vi "Do.vi"(8 "error in (no error)":errorcluster, 10 "Actor in":refnum<class "Actor.lvclass">, 11 "Trace Query Options Msg":refnum<class "Trace Query Options Msg.lvclass">) -> (0 "error out":errorcluster, 2 "Actor out":refnum<class "Actor.lvclass">)   [LabVIEW 2017, in "BNT_DSCXtGraph.lvlib" / "Trace Query Options Msg.lvclass"]
doc: "This VI delivers the message to the actor by calling the appropriate method(s) on the actor."
uses:
  Trace Query Options Msg.lvclass
  <vilib>/ActorFramework/Actor/Actor.lvclass
  BNT_DSCXtGraph/BNT_DSCXtGraph.lvclass
  C:/Program Files (x86)/National Instruments/LabVIEW 2017/vi.lib/ActorFramework/Actor/Actor.lvclass
  Trace Query Options Msg.lvclass/Trace Query Options Msg.ctl
  CSPP_Core/Messages/CSPP_AsyncCallbackMsg/CSPP_AsyncCallback Msg.lvclass
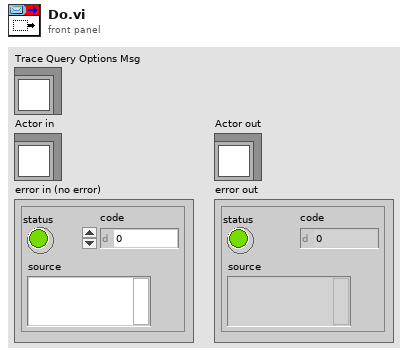
[diagram p1: front panel]
types:
  T1 = cluster{"Start Time":timestamp, "Stop Time":timestamp}
  T2 = cluster{"interpolate data (F)":bool, "extrapolate to now (F)":bool, "remove data breaks (F)":bool, "interpolation interval (1 s)":dbl, "maintain trending info (T)":bool}
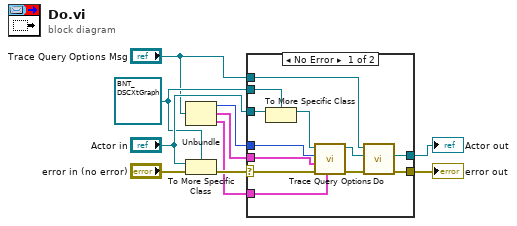
[diagram p0: block diagram]
diagram:
  w5 = refnum<class "BNT_DSCXtGraph.lvclass"> refnum ("Actor in")
  n1 = Unbundle ("Main-Unbundler")("Trace Query Options Msg") -> (w3:i32, w2:T1, w1:T2)
  n2 = To More Specific Class(target class=w5, reference="Actor in", error in="error in (no error)") -> (error out=w9:errorcluster)  [unwired: 1 out]
  n3 = case shown="No Error" w9 {
    selector: w9 -> [w22 w24]
    tunnel: [w19 w24] -> w8
    tunnel: [w18 w23] -> w7
    tunnel: "Actor in" -> [w21 w23]
    tunnel: w5 -> [w20 _]
    tunnel: "Trace Query Options Msg" -> [w16 _]
    tunnel: w3 -> [w13 _]
    tunnel: w2 -> [w12 _]
    tunnel: w1 -> [w11 _]
    frame No Error {
      n4 = To More Specific Class ("To More Specific Class (internal)")(target class=w20, reference=w21) -> (specific class reference=w15:refnum<class "BNT_DSCXtGraph.lvclass">)  [unwired: 1 in, 1 out]
      n5 = call "Trace Query Options.vi"("Options"=w11, "Error In"=w22, "Time Interval"=w12, "Max Points per Trace (all)"=w13, "BNT_DSCXtGraph in"=w15) -> ("Error Out"=w17:errorcluster, "BNT_DSCXtGraph out"=w14:refnum<class "BNT_DSCXtGraph.lvclass">)  [unwired: 5 in]
      n6 = call-parent "Do.vi"("error in (no error)"=w17, "Actor in"=w14, "CSPP_AsyncCallback Msg"=w16) -> ("error out"=w19:errorcluster, "Actor out"=w18:refnum<class "Actor.lvclass">)  [unwired: 7 in]
    }
    frame Error {
    }
  }
  "error out" <- w8
  "Actor out" <- w7
